vi "Vision Processing.vi"() -> ()   [LabVIEW 2011]
doc: "This VI runs in parallel to other tasks. It gets images from the camera, processes them for color or shape and use that information to affect robot behavior."
uses:
  <vilib>/Rock Robotics/WPI/Camera/WPI_CameraImageSize.ctl
  <vilib>/Rock Robotics/WPI/Camera/WPI_CameraWhite Balance Values.ctl
  Robot Global Data.vi
  <vilib>/vision/NI_Vision_Development_Module.lvlib
panel:
  in  "Range":cluster{"Lower value":sgl, "Upper value":sgl}={"Lower value"=120.0, "Upper value"=255.0}
  out "RightMotor":bool
  in  "Motor Limit":dbl=0.5
  out "LeftMotor":bool
  out "Motor Output":dbl
  in  "Camera Settings":T2={"FPS"=15, "Compression"=30, "Image Size"=enum."160x120"}
  in  "Camera IP Address":string="10.0.27.11"
  out "Processed Image":T3(plugin-control)
  out "Original Image":T3(plugin-control)
  in  "Annotate":bool=TRUE
  in  "Particle Count Limit":i32=10
  in  "Area Size Limit":i32=444
  in  "Camera Type":enum16{"206", "1011"}(ring)=enum."1011"
  out "output cluster":T4
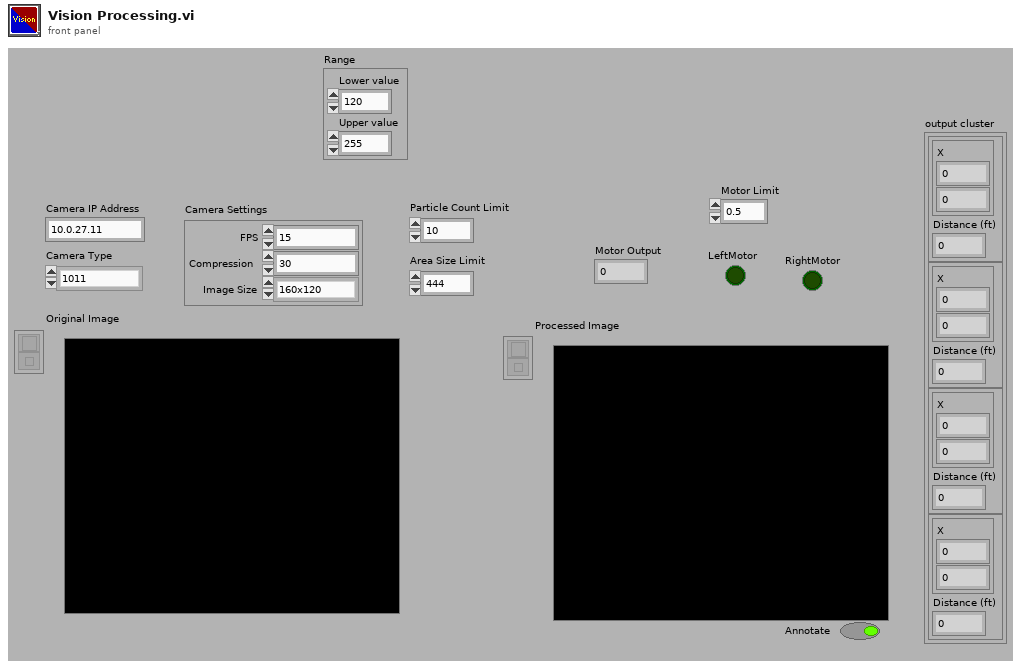
[diagram p1: front panel]
types:
  T1 = typedef "WPI_CameraImageSize.ctl" = enum16{"640x480", "320x240", "160x120"}
  T2 = cluster{"FPS":i32, "Compression":i32, "Image Size":T1}
  T3 = typedef "IMAQ Image.ctl" = refnum<image>
  T4 = cluster{cluster{cluster{"X":dbl, dbl}, "Distance (ft)":dbl}, cluster{cluster{"X":dbl, dbl}, "Distance (ft)":dbl}, cluster{cluster{"X":dbl, dbl}, "Distance (ft)":dbl}, cluster{cluster{"X":dbl, dbl}, "Distance (ft)":dbl}}
  T5 = typedef "WPI_CameraWhite Balance Values.ctl" = enum16{"Auto", "Fixed indoor", "Fixed outdoor 1", "Fixed outdoor 2", "Fixed fluorescent 1", "Fixed fluorescent 2", "Hold current"}
  T6 = typedef "Image Type" = u32
  T7 = typedef "WPI_CameraDevRef.ctl" = cluster{"Camera Address":string, "CameraStatus":errorcluster, "Acquire Image Notifier":refnum<notifier>}
  T8 = cluster{"Rect Coverage":dbl, "Aspect Ratio":dbl, "X Edge Strength":dbl, "Y Edge Strength":dbl}
  T9 = cluster{"Position":cluster{"X":dbl, "Y":dbl}, "Distance (ft)":dbl}[]
  T10 = cluster{cluster{"Left":dbl, "Top":dbl, "Right":dbl, "Bottom":dbl}, dbl[]}[]
  T11 = cluster{"Left":dbl, "Top":dbl, "Right":dbl, "Bottom":dbl}
  T12 = cluster{"Target Center (-1 to 1)":cluster{"X":dbl, "Y":dbl}, "Distance (ft)":dbl}
  T13 = cluster{"Target Center (-1 to 1)":cluster{"X":dbl, "Y":dbl}, "Distance (ft)":dbl}[]
  T14 = cluster{"Position":cluster{"X":dbl, "Y":dbl}, "Distance (ft)":dbl}
  T15 = cluster{cluster{"X":dbl, dbl}, "Distance (ft)":dbl}
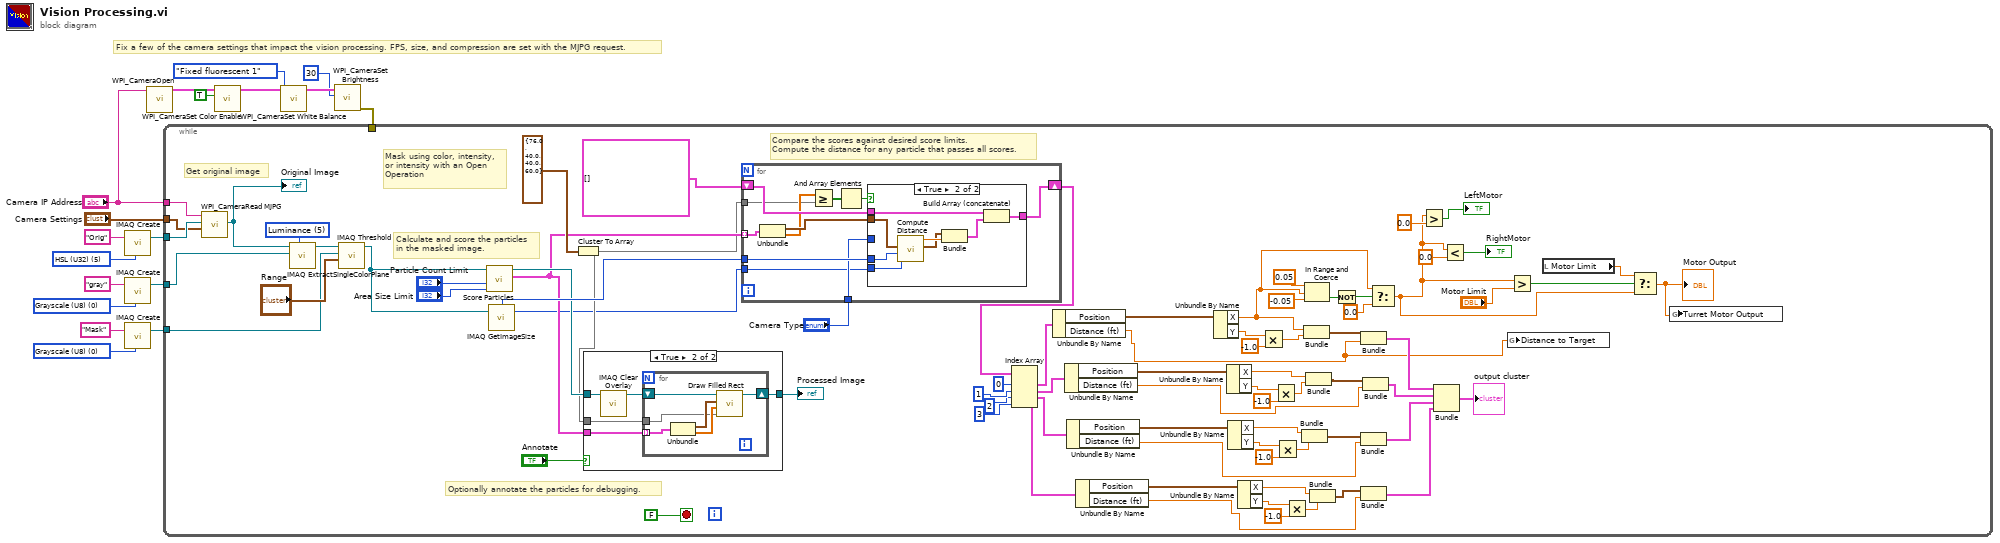
[diagram p0: block diagram]
diagram:
  w11 = T6 0 items=["Grayscale (U8)", "Grayscale (I16)", "Grayscale (SGL)", "Complex (CSG)", "RGB (U32)", "HSL (U32)", "RGB (U64)", "Grayscale (U16)"] ("Image Type")
  w15 = T6 5 items=["Grayscale (U8)", "Grayscale (I16)", "Grayscale (SGL)", "Complex (CSG)", "RGB (U32)", "HSL (U32)", "RGB (U64)", "Grayscale (U16)"] ("Image Type")
  w18 = T6 0 items=["Grayscale (U8)", "Grayscale (I16)", "Grayscale (SGL)", "Complex (CSG)", "RGB (U32)", "HSL (U32)", "RGB (U64)", "Grayscale (U16)"] ("Image Type")
  # "Fix a few of the camera settings that impact the vision processing. FPS, size, and compression are set with the MJPG request."
  n1 = call "IMAQ Create"("Image Name"="Orig", "Image Type"=w15) -> ("New Image"=w14:T3)  [unwired: 2 in, 2 out]
  n2 = call "IMAQ Create"("Image Name"="gray", "Image Type"=w18) -> ("New Image"=w13:T3)  [unwired: 2 in, 2 out]
  n3 = call "IMAQ Create"("Image Name"="Mask", "Image Type"=w11) -> ("New Image"=w10:T3)  [unwired: 2 in, 2 out]
  n4 = call <vilib>:"WPI_CameraOpen.vi"("Camera Address"="Camera IP Address") -> ("CameraDevRef"=w8:T7)  [unwired: 9 in, 1 out]
  n5 = call <vilib>:"WPI_CameraSet Color Enable.vi"("Color Enabled"=TRUE, "CameraDevRef"=w8) -> ("CameraDevRef Out"=w6:T7)  [unwired: 8 in, 1 out]
  n6 = call <vilib>:"WPI_CameraSet White Balance.vi"("White Balance"=WPI_CameraWhite_Balance_Values."Fixed fluorescent 1", "CameraDevRef"=w6) -> ("CameraDevRef Out"=w4:T7)  [unwired: 8 in, 1 out]
  n7 = call <vilib>:"WPI_CameraSet Brightness.vi"("Brightness"=30, "CameraDevRef"=w4) -> ("error out"=w2:errorcluster)  [unwired: 8 in, 1 out]
  n8 = while {
    tunnel: w14 -> [w95]
    tunnel: w13 -> [w37]
    tunnel: w10 -> [w39]
    tunnel: "Camera IP Address" -> [w94]
    tunnel: w2 -> [_]
    tunnel: "Camera Settings" -> [w82]
    stop <- FALSE stop-if-true
    w42 = 5 items=["Red", "Green", "Blue", "Hue", "Saturation", "Luminance", "Value", "Intensity"] ("Color Plane")
    # "Optionally annotate the particles for debugging."
    # "Compare the scores against desired score limits.\nCompute the distance for any particle that passes all scores."
    # "Calculate and score the particles\nin the masked image."
    # "Mask using color, intensity,\nor intensity with an Open\nOperation"
    # "Get original image"
    n9 = call <vilib>:"WPI_CameraRead MJPG.vi"("Camera Settings"=w82, "Image"=w95, "address"=w94) -> ("Image Out"=w38:T3)  [unwired: 7 in, 1 out]
    "Original Image" <- w38
    n10 = call "IMAQ ExtractSingleColorPlane"("Color Plane"=w42, "Image Dst"=w37, "Image Src"=w38) -> ("Image Dst Out"=w40:T3)  [unwired: 1 in, 7 out]
    n11 = call "IMAQ Threshold"("Range"="Range", "Image Dst"=w39, "Image Src"=w40) -> ("Image Dst Out"=w36:T3)  [unwired: 3 in, 5 out]
    n12 = call "Score Particles.vi"("Area Size Limit"="Area Size Limit", "Particle Count Limit"="Particle Count Limit", "Image Refnum in"=w36) -> ("Scored Particle Info"=w89:T10, "Image Refnum out"=w93:T3)  [unwired: 7 in]
    n13 = call "IMAQ GetImageSize"("Image"=w36) -> ("Y Resolution"=w83:i32, "X Resolution"=w96:i32)  [unwired: 3 in, 1 out]
    n14 = Cluster To Array(cluster=T8 {"Rect Coverage"=76.0, "Aspect Ratio"=40.0, "X Edge Strength"=40.0, "Y Edge Strength"=60.0} ("Score Limits")) -> (array=w87:dbl[])
    n15 = case shown="True" "Annotate" {
      tunnel: w93 -> [w98 w103]
      tunnel: [w98 w102] -> w90
      tunnel: w89 -> [_ w100]
      tunnel: w87 -> [_ w99]
      frame False {
      }
      frame True {
        n16 = call "IMAQ Clear Overlay"("Image"=w103) -> ("Image Out"=w101:T3)  [unwired: 2 in, 8 out]
        n17 = for {
          shift-right: [w108] -> w102
          shift-left: w101 -> [w109]
          tunnel: w100 -> [w105] mode=indexing
          tunnel: w99 -> [w104]
          n18 = Unbundle(w105) -> (w106:T11, w107:dbl[])
          n19 = call "Draw Filled Rect.vi"("Limits"=w104, "Scores"=w107, "Bounding Box"=w106, "image in"=w109) -> ("image out"=w108:T3)  [unwired: 7 in]
        }
      }
    }
    "Processed Image" <- w90
    n20 = for {
      shift-right: [w119] -> w30
      shift-left: T9 [] -> [w120]
      tunnel: w96 -> [w118]
      tunnel: w89 -> [w116] mode=indexing
      tunnel: w87 -> [w111]
      tunnel: "Camera Type" -> [w115]
      tunnel: w83 -> [w110]
      n21 = Unbundle(w116) -> (w117:T11, w112:dbl[])
      n22 = Greater Or Equal?(x=w112, y=w111) -> (x >= y?=w114:bool[])
      n23 = And Array Elements(Boolean array=w114) -> (logical AND=w113:bool)
      n24 = case shown="True" w113 {
        tunnel: w120 -> [w121 w129]
        tunnel: [w121 w128] -> w119
        tunnel: w117 -> [_ w124]
        tunnel: w118 -> [_ w126]
        tunnel: w115 -> [_ _]
        tunnel: w110 -> [_ w122]
        frame False {
        }
        frame True {
          n25 = call "Compute Distance.vi"("Y Image Resolution"=w122, "X Image Resolution"=w126, "Bounding Box"=w124) -> ("Target Center (-1 to 1)"=w123:cluster{"X":dbl, "Y":dbl}, "Distance (ft)"=w125:dbl)  [unwired: 7 in]
          n26 = Bundle("Target Center (-1 to 1)"=w123, "Distance (ft)"=w125) -> (w127:T12)  [unwired: 1 in]
          n27 = Build Array (concatenate)(w129, w127) -> (w128:T13)
        }
      }
    }
    n28 = Index Array(array=w30, index #1=0 ("index"), index #2=1 ("index"), index #3=2 ("index"), index #4=3 ("index")) -> (element #1=w77:T14, element #2=w64:T14, element #3=w63:T14, element #4=w62:T14)
    n29 = Unbundle By Name(w77) -> ("Position"=w76:cluster{"X":dbl, "Y":dbl}, "Distance (ft)"=w19:dbl)
    n30 = Unbundle By Name(w64) -> ("Position"=w71:cluster{"X":dbl, "Y":dbl}, "Distance (ft)"=w59:dbl)
    n31 = Unbundle By Name(w63) -> ("Position"=w70:cluster{"X":dbl, "Y":dbl}, "Distance (ft)"=w58:dbl)
    n32 = Unbundle By Name(w62) -> ("Position"=w65:cluster{"X":dbl, "Y":dbl}, "Distance (ft)"=w48:dbl)
    n33 = Unbundle By Name(w76) -> ("X"=w22:dbl, "Y"=w74:dbl)
    n34 = Unbundle By Name(w71) -> ("X"=w57:dbl, "Y"=w73:dbl)
    n35 = Unbundle By Name(w70) -> ("X"=w54:dbl, "Y"=w68:dbl)
    n36 = Unbundle By Name(w65) -> ("X"=w51:dbl, "Y"=w67:dbl)
    n37 = Multiply(x=w74, y=-1.0 ("x")) -> (x*y=w61:dbl)
    n38 = Multiply(x=w73, y=-1.0 ("x")) -> (x*y=w56:dbl)
    n39 = Multiply(x=w68, y=-1.0 ("x")) -> (x*y=w53:dbl)
    n40 = Multiply(x=w67, y=-1.0 ("x")) -> (x*y=w50:dbl)
    n41 = Bundle("X"=w54, w53) -> (w52:cluster{"X":dbl, dbl})  [unwired: 1 in]
    n42 = Bundle("X"=w22, w61) -> (w60:cluster{"X":dbl, dbl})  [unwired: 1 in]
    n43 = In Range and Coerce(upper limit=0.05, x=w22, lower limit=-0.05) -> (In Range?=w33:bool)  [unwired: 1 out]
    n44 = Bundle("X"=w57, w56) -> (w55:cluster{"X":dbl, dbl})  [unwired: 1 in]
    n45 = Bundle("X"=w51, w50) -> (w49:cluster{"X":dbl, dbl})  [unwired: 1 in]
    n46 = Not(x=w33) -> (.not. x?=w32:bool)
    n47 = Bundle(w52, "Distance (ft)"=w58) -> (w45:T15)  [unwired: 1 in]
    n48 = Bundle(w49, "Distance (ft)"=w48) -> (w44:T15)  [unwired: 1 in]
    n49 = Bundle(w60, "Distance (ft)"=w19) -> (w47:T15)  [unwired: 1 in]
    n50 = Bundle(w55, "Distance (ft)"=w59) -> (w46:T15)  [unwired: 1 in]
    n51 = Select(t=w22, s=w32, f=0.0) -> (s? t:f=w24:dbl)
    n52 = Greater?(x=w24, y=0.0) -> (0:→"LeftMotor":bool)
    n53 = Bundle(w47, w46, w45, w44) -> (→"output cluster":T4)  [unwired: 1 in]
    n54 = Less?(x=w24, y=0.0) -> (x < y?=→"RightMotor":bool)
    n55 = global write "Robot Global Data.vi" "Distance to Target"(w19) -> ()
    n56 = Greater?(x=w24, y="Motor Limit") -> (0:w27:bool)
    n57 = local read "Motor Limit"() -> (w26:dbl)
    n58 = Select(t=w26, s=w27, f=w24) -> (s? t:f=w25:dbl)
    "Motor Output" <- w25
    n59 = global write "Robot Global Data.vi" "Turret Motor Output"(w25) -> ()
  }
